vi "ILD from Array Data.vi"(8 "Frequency":dbl[](array[numeric]), 9 "Data in":dbl[](array[numeric]), 11 "Spec":enum16{"IEEE802.3ba", "FDR", "EDR"}(ring)) -> (0 "Size":i32, 1 "ILD Data":dbl[](array[numeric]), 2 "ILD":cluster{"all rows":dbl[], sgl[]}[](graph), 3 "IL Fitted":cluster{"all rows":dbl[], "IL":dbl[]}[](graph))   [LabVIEW 2011]
uses:
  <vilib>/Analysis/baseanly.llb/Real A x B.vi
  <vilib>/Analysis/baseanly.llb/Real Inverse Matrix.vi
  <vilib>/Analysis/baseanly.llb/A x Vector.vi
  <vilib>/Analysis/NI_AALBase.lvlib
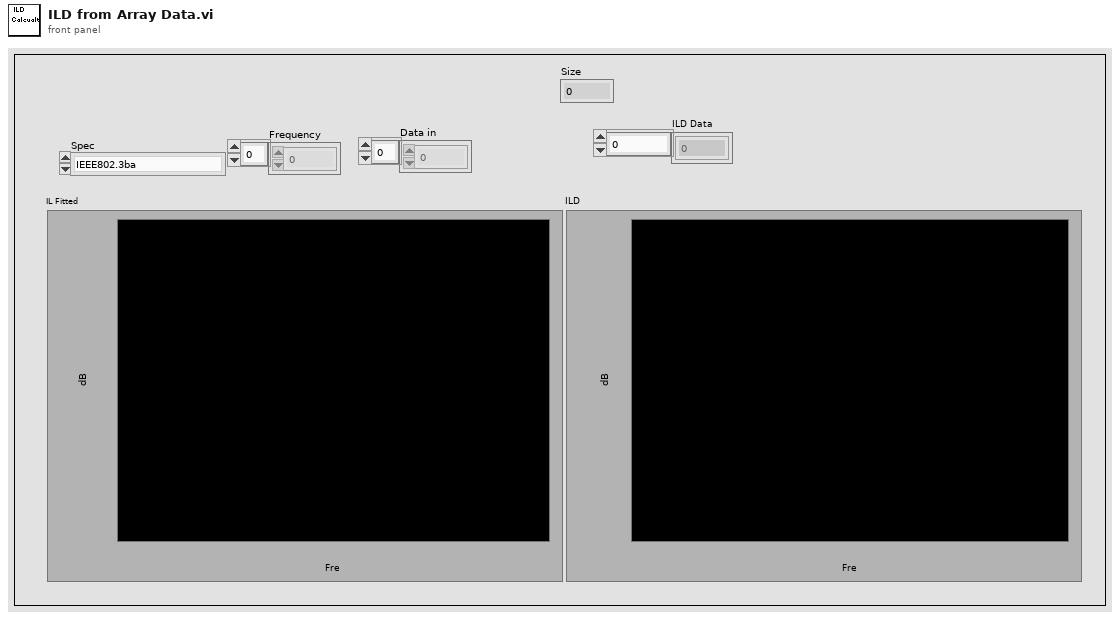
[diagram p1: front panel]
types:
  T1 = typedef "NI_Matrix.lvlib/RealMatrix.ctl" = dbl[][]
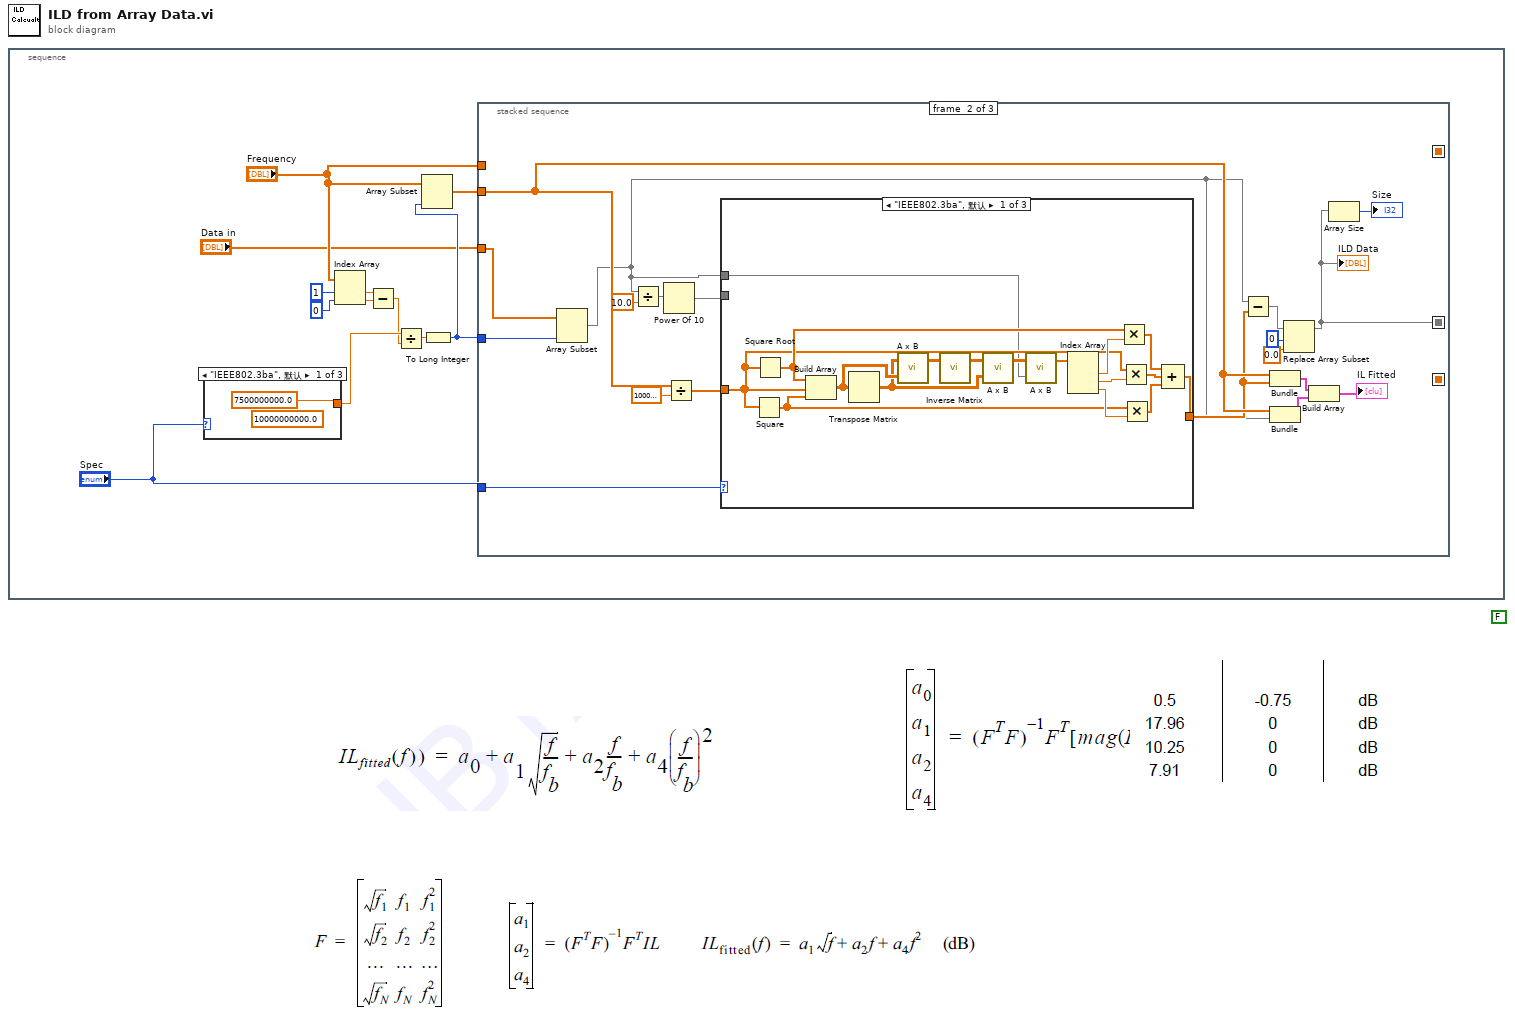
[diagram p0: block diagram]
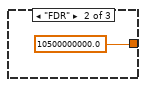
[diagram p2: hidden frame]
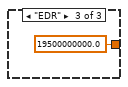
[diagram p3: hidden frame]
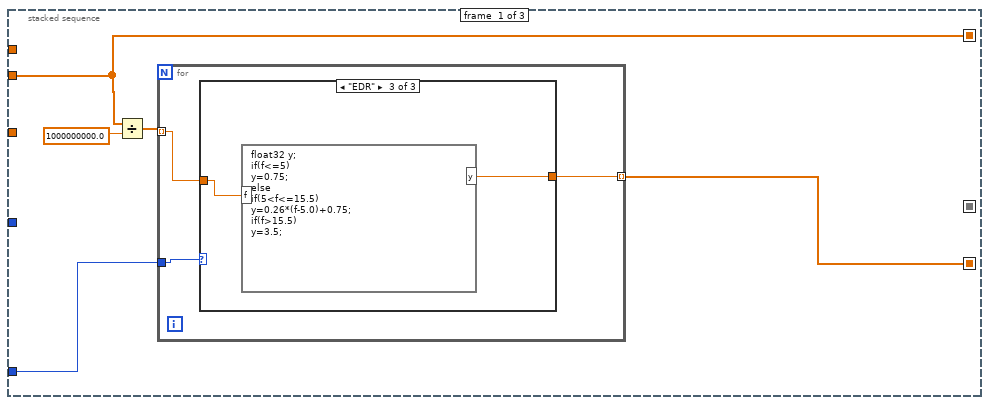
[diagram p4: hidden frame]
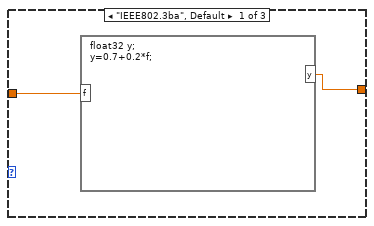
[diagram p5: hidden frame]
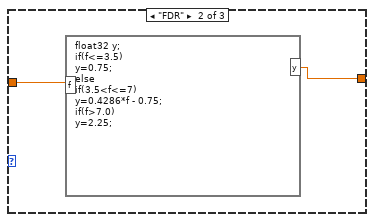
[diagram p6: hidden frame]
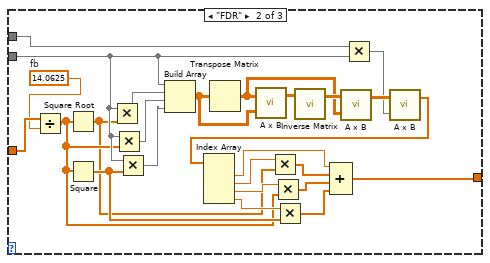
[diagram p7: hidden frame]
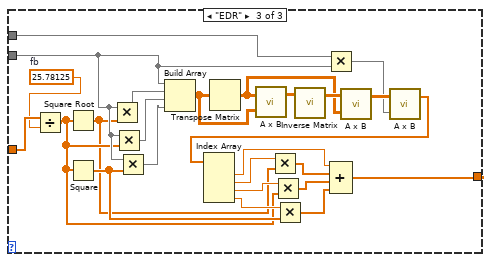
[diagram p8: hidden frame]
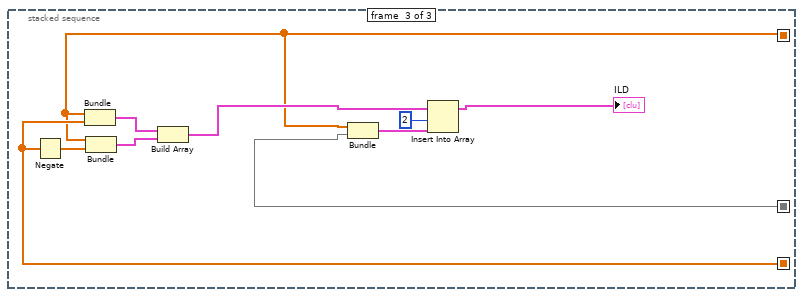
[diagram p9: hidden frame]
diagram:
  (unwired) FALSE
  n1 = stacked-sequence {
    frame #0 {
      n2 = case shown="\"IEEE802.3ba\", 默认" "Spec" {
        tunnel: [7500000000.0 ("y") 10500000000.0 ("y") 19500000000.0 ("y")] -> w9
        frame "IEEE802.3ba", Default {
          (unwired) 10000000000.0 ("y")
        }
        frame "FDR" {
        }
        frame "EDR" {
        }
      }
      n3 = Index Array(array="Frequency", index #1=1 ("索引"), index #2=0 ("索引")) -> (element #1=w7:dbl, element #2=w8:dbl)
      n4 = Subtract(x=w7, y=w8) -> (x-y=w6:dbl)
      n5 = Divide(x=w9, y=w6) -> (x/y=w5:dbl)
      n6 = To Long Integer(number=w5) -> (32bit integer=w3:i32)
      n7 = Array Subset(array="Frequency", length=w3) -> (w4:dbl[])  [unwired: 1 in]
      n8 = stacked-sequence {
        seq-local: [w19 _ _] -> [_ _ w123]
        seq-local: [w16 _ _] -> [_ _ w119]
        seq-local: [_ w31 _] -> [_ _ w120]
        tunnel: "Spec" -> [w20 w48 _]
        tunnel: w4 -> [w16 w47 _]
        tunnel: w3 -> [_ w46 _]
        tunnel: "Frequency" -> [_ _ _]
        tunnel: "Data in" -> [_ w45 _]
        frame #0 {
          n9 = Divide(x=w16, y=1000000000.0) -> (x/y=w18:dbl[])
          n10 = for {
            tunnel: w20 -> [w23]
            tunnel: w18 -> [w22] mode=indexing
            tunnel: [w21] -> w19 mode=indexing
            n11 = case shown="\"EDR\"" w23 {
              tunnel: w22 -> [w25 w27 w29]
              tunnel: [w24 w26 w28] -> w21
              frame "IEEE802.3ba", Default {
                n12 = formula code="float32 y;\ny=0.7+0.2*f;"("f"=w25) -> ("y"=w24:sgl)
              }
              frame "FDR" {
                n13 = formula code="float32 y;\nif(f<=3.5)\ny=0.75;\nelse\nif(3.5<f<=7)\ny=0.4286*f - 0.75;\nif(f>7.0)\ny=2.25;"("f"=w27) -> ("y"=w26:sgl)
              }
              frame "EDR" {
                n14 = formula code="float32 y;\nif(f<=5)\ny=0.75;\nelse\nif(5<f<=15.5)\ny=0.26*(f-5.0)+0.75;\nif(f>15.5)\ny=3.5;"("f"=w29) -> ("y"=w28:sgl)
              }
            }
          }
        }
        frame #1 {
          n15 = Array Subset(array=w45, length=w46) -> (w32:dbl[])  [unwired: 1 in]
          n16 = Divide(x=w32, y=10.0 ("新元素/子数组")) -> (x/y=w35:dbl[])
          n17 = Power Of 10(x=w35) -> (10^x=w34:dbl[])
          n18 = Divide(x=w47, y=1000000000.0) -> (x/y=w33:dbl[])
          n19 = case shown="\"IEEE802.3ba\", 默认" w48 {
            tunnel: [w51 w66 w91] -> w40
            tunnel: w33 -> [w50 w90 w115]
            tunnel: w32 -> [w49 w80 w105]
            tunnel: w34 -> [_ w79 w104]
            frame "IEEE802.3ba", Default {
              n20 = Square(x=w50) -> (x^2=w55:dbl[])
              n21 = Square Root(x=w50) -> (sqrt(x)=w56:dbl[])
              n22 = Build Array(w56, w50, w55) -> (w65:T1)
              n23 = Transpose Matrix(1:w65) -> (0:w63:T1)
              n24 = call-poly <vilib>:"A x B.vi"("B"=w65, "A"=w63) -> ("A x B"=w64:T1)  [unwired: 1 out]
              n25 = call-poly <vilib>:"Inverse Matrix.vi"("Input Matrix"=w64) -> ("Inverse Matrix"=w62:T1)  [unwired: 1 in, 1 out]
              n26 = call-poly <vilib>:"A x B.vi"("B"=w63, "A"=w62) -> ("A x B"=w61:T1)  [unwired: 1 out]
              n27 = call-poly <vilib>:"A x B.vi"("Vector"=w49, "A"=w61) -> ("A x Vector"=w60:dbl[])  [unwired: 1 out]
              n28 = Index Array(array=w60) -> (element #1=w57:dbl, element #2=w58:dbl, element #3=w59:dbl)  [unwired: 3 in]
              n29 = Multiply(x=w56, y=w57) -> (x*y=w54:dbl[])
              n30 = Multiply(x=w50, y=w58) -> (x*y=w53:dbl[])
              n31 = Multiply(x=w55, y=w59) -> (x*y=w52:dbl[])
              n32 = Compound Arithmetic op=ADD(w54, w53, w52) -> (w51:dbl[])
            }
            frame "FDR" {
              w89 = 14.0625  # fb
              n33 = Divide(x=w90, y=w89) -> (x/y=w68:dbl[])
              n34 = Square Root(x=w68) -> (sqrt(x)=w67:dbl[])
              n35 = Square(x=w68) -> (x^2=w69:dbl[])
              n36 = Multiply(x=w79, y=w67) -> (x*y=w88:dbl[])
              n37 = Multiply(x=w79, y=w68) -> (x*y=w87:dbl[])
              n38 = Multiply(x=w79, y=w69) -> (x*y=w86:dbl[])
              n39 = Build Array(w79, w88, w87, w86) -> (w85:T1)
              n40 = Transpose Matrix(1:w85) -> (0:w82:T1)
              n41 = call-poly <vilib>:"A x B.vi"("B"=w85, "A"=w82) -> ("A x B"=w84:T1)  [unwired: 1 out]
              n42 = call-poly <vilib>:"Inverse Matrix.vi"("Input Matrix"=w84) -> ("Inverse Matrix"=w83:T1)  [unwired: 1 in, 1 out]
              n43 = call-poly <vilib>:"A x B.vi"("B"=w82, "A"=w83) -> ("A x B"=w81:T1)  [unwired: 1 out]
              n44 = Multiply(x=w80, y=w79) -> (x*y=w78:dbl[])
              n45 = call-poly <vilib>:"A x B.vi"("Vector"=w78, "A"=w81) -> ("A x Vector"=w77:dbl[])  [unwired: 1 out]
              n46 = Index Array(array=w77) -> (element #1=w76:dbl, element #2=w75:dbl, element #3=w74:dbl, element #4=w73:dbl)  [unwired: 4 in]
              n47 = Multiply(x=w75, y=w67) -> (x*y=w72:dbl[])
              n48 = Multiply(x=w74, y=w68) -> (x*y=w71:dbl[])
              n49 = Multiply(x=w73, y=w69) -> (x*y=w70:dbl[])
              n50 = Compound Arithmetic op=ADD(w76, w72, w71, w70) -> (w66:dbl[])
            }
            frame "EDR" {
              w114 = 25.78125  # fb
              n51 = Divide(x=w115, y=w114) -> (x/y=w93:dbl[])
              n52 = Square Root(x=w93) -> (sqrt(x)=w92:dbl[])
              n53 = Square(x=w93) -> (x^2=w94:dbl[])
              n54 = Multiply(x=w104, y=w92) -> (x*y=w113:dbl[])
              n55 = Multiply(x=w104, y=w93) -> (x*y=w112:dbl[])
              n56 = Multiply(x=w104, y=w94) -> (x*y=w111:dbl[])
              n57 = Build Array(w104, w113, w112, w111) -> (w110:T1)
              n58 = Transpose Matrix(1:w110) -> (0:w107:T1)
              n59 = call-poly <vilib>:"A x B.vi"("B"=w110, "A"=w107) -> ("A x B"=w109:T1)  [unwired: 1 out]
              n60 = call-poly <vilib>:"Inverse Matrix.vi"("Input Matrix"=w109) -> ("Inverse Matrix"=w108:T1)  [unwired: 1 in, 1 out]
              n61 = Multiply(x=w105, y=w104) -> (x*y=w103:dbl[])
              n62 = call-poly <vilib>:"A x B.vi"("B"=w107, "A"=w108) -> ("A x B"=w106:T1)  [unwired: 1 out]
              n63 = call-poly <vilib>:"A x B.vi"("Vector"=w103, "A"=w106) -> ("A x Vector"=w102:dbl[])  [unwired: 1 out]
              n64 = Index Array(array=w102) -> (element #1=w101:dbl, element #2=w100:dbl, element #3=w99:dbl, element #4=w98:dbl)  [unwired: 4 in]
              n65 = Multiply(x=w100, y=w92) -> (x*y=w97:dbl[])
              n66 = Multiply(x=w99, y=w93) -> (x*y=w96:dbl[])
              n67 = Multiply(x=w98, y=w94) -> (x*y=w95:dbl[])
              n68 = Compound Arithmetic op=ADD(w101, w97, w96, w95) -> (w91:dbl[])
            }
          }
          n69 = Subtract(x=w32, y=w40) -> (x-y=w39:dbl[])
          n70 = Bundle(w47, w40) -> (w44:cluster{dbl[], dbl[]})  [unwired: 1 in]
          n71 = Bundle(w47, w32) -> (w43:cluster{dbl[], dbl[]})  [unwired: 1 in]
          n72 = Replace Array Subset(array=w39, new element=0.0 ("新元素/子数组"), index=0 ("索引")) -> (w31:dbl[])
          "ILD Data" <- w31
          n73 = Build Array(w44, w43) -> (→"IL Fitted":cluster{dbl[], dbl[]}[])
          n74 = Array Size(array=w31) -> (size(s)=→"Size":i32)
        }
        frame #2 {
          n75 = Negate(x=w123) -> (-x=w124:sgl[])
          n76 = Bundle(w119, w123) -> (w122:cluster{dbl[], sgl[]})  [unwired: 1 in]
          n77 = Bundle(w119, w124) -> (w125:cluster{dbl[], sgl[]})  [unwired: 1 in]
          n78 = Build Array(w122, w125) -> (w121:cluster{dbl[], sgl[]}[])
          n79 = Bundle(w119, w120) -> (w117:cluster{dbl[], dbl[]})  [unwired: 1 in]
          n80 = Insert Into Array(array=w121, index=2 ("y"), new element=w117) -> (→"ILD":cluster{dbl[], sgl[]}[])
        }
      }
    }
  }
